vi "Add Array Data Channels.vi"(8 "Error In":errorcluster, 10 "Array Elements":T2[](array[typedef]), 11 "Section Refnum In":T1 format="%.0x") -> (0 "Error Out":errorcluster, 3 "Channel Refnums":T1[](array[typedef]) format="%.0x")   [LabVIEW 2018, in "Instrument Addon System Explorer.lvlib"]
doc: "Adds channels under the Data Array section provided as reference input."
uses:
  Instrument Addon System Explorer.lvlib
  <vilib>/NI Veristand/Custom Device API/Custom Device Item Ref.ctl
  APIs/Scripting API/TypeDefs/Array Element.ctl
  <vilib>/NI Veristand/Custom Device API/Custom Device Channel.ctl
  <vilib>/NI Veristand/Custom Device API/Custom Device Channel Type.ctl
  Addon Shared/SubVIs/Constants.vi
  Addon Shared/Instrument Addon Shared.lvlib
  <vilib>/NI Veristand/Custom Device API/Custom Device API.lvlib
  APIs/Scripting API/Instrument Addon Scripting API.lvlib
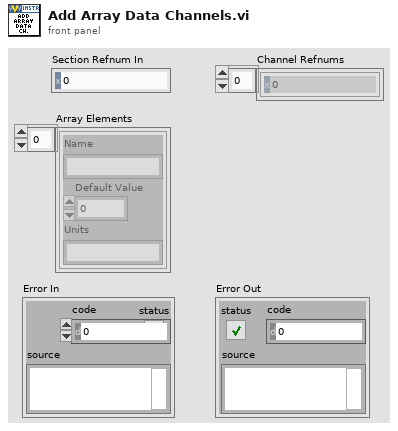
[diagram p1: front panel]
types:
  T1 = typedef "Custom Device API.lvlib/Custom Device Item Ref.ctl" = u64
  T2 = typedef "Instrument Addon Scripting API.lvlib/Array Element.ctl" = cluster{"Name":string, "Default Value":dbl, "Units":string}
  T3 = typedef "Custom Device API.lvlib/Custom Device Channel.ctl" = cluster{"Type":T4, "Units":string, "Default Value":dbl, "Faultable":bool, "Scalable":bool}
  T4 = typedef "Custom Device API.lvlib/Custom Device Channel Type.ctl" = enum16{"Input", "Output"}
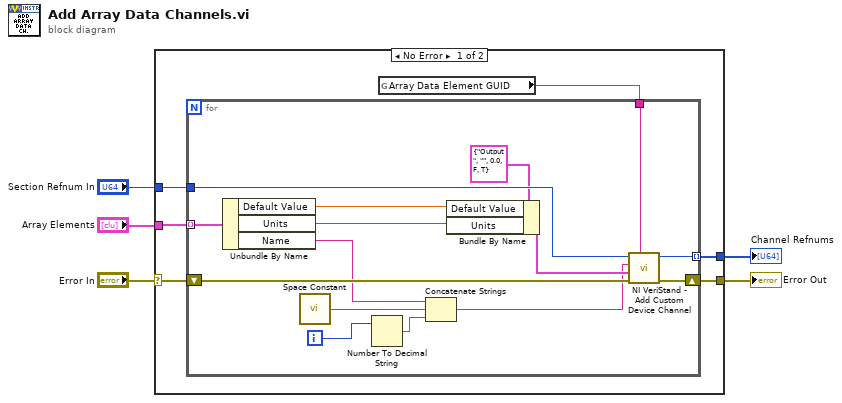
[diagram p0: block diagram]
diagram:
  n1 = case shown="No Error" "Error In" {
    selector: "Error In" -> [w8 w27]
    tunnel: [w11 w27] -> w5
    tunnel: "Section Refnum In" -> [w10 _]
    tunnel: "Array Elements" -> [w6 _]
    tunnel: [w7 _] -> w1
    frame No Error {
      n2 = global read "Constants.vi" "Array Data Element GUID"() -> (w9:string)
      n3 = for {
        shift-right: [w26] -> w11
        shift-left: w8 -> [w20]
        tunnel: w9 -> [w25]
        tunnel: w10 -> [w19]
        tunnel: w6 -> [w24] mode=indexing
        tunnel: [w21] -> w7 mode=indexing
        i -> [w17]
        n4 = Unbundle By Name(w24) -> ("Default Value"=w23:dbl, "Units"=w22:string, "Name"=w18:string)
        n5 = call <vilib>:"Space Constant.vi"() -> ("String"=w14:string)
        n6 = Number To Decimal String(number=w17) -> (decimal integer string=w13:string)  [unwired: 1 in]
        n7 = Concatenate Strings(w18, w14, w13) -> (w12:string)
        n8 = Bundle By Name(cluster=T3 {"Type"=enum."Output", "Units"="", "Default Value"=0.0, "Faultable"=FALSE, "Scalable"=TRUE} ("Channel"), "Default Value"=w23, "Units"=w22) -> (w15:T3)
        n9 = call <vilib>:"NI VeriStand - Add Custom Device Channel.vi"("GUID (Default Channel)"=w25, "error in (no error)"=w20, "Channel"=w15, "Channel Name"=w12, "Parent Ref in"=w19) -> ("error out"=w26:errorcluster, "Parent Ref out"=w21:T1)  [unwired: 3 in, 2 out]
      }
    }
    frame Error {
    }
  }
  "Error Out" <- w5
  "Channel Refnums" <- w1
